vi "create_folder_general-SD.vi"(2 "error in (no error)":errorcluster, 3 "save Radio Buttons":enum32{"Automatic", "User-def"}(ring), 4 "Name":string) -> (0 "error out":errorcluster, 1 "appended path":path)   [LabVIEW 2020]
uses:
  globalVarSD.vi
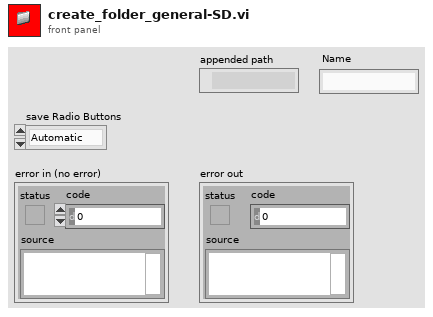
[diagram p1: front panel]
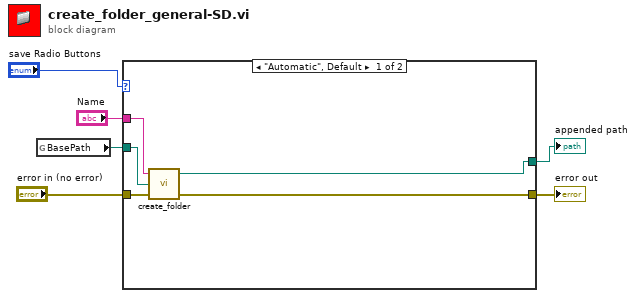
[diagram p0: block diagram]
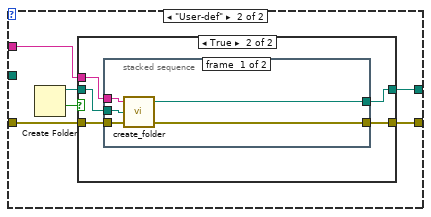
[diagram p2: hidden frame]
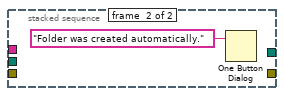
[diagram p4: hidden frame]
diagram:
  n1 = global read "globalVarSD.vi" "BasePath"() -> (w1:path)
  n2 = case shown="\"Automatic\", Default" "save Radio Buttons" {
    tunnel: [w11 w14] -> w2
    tunnel: w1 -> [w8 _]
    tunnel: "error in (no error)" -> [w10 w16]
    tunnel: [w9 w15] -> w5
    tunnel: "Name" -> [w7 w12]
    frame "Automatic", Default {
      n3 = call "create_folder.vi"("Name"=w7, "base path"=w8, "error in"=w10) -> ("appended path"=w11:path, "error out"=w9:errorcluster)  [unwired: 5 in]
    }
    frame "User-def" {
      n4 = Create Folder() -> (created path=w13:path, cancelled=w17:bool)  [unwired: 3 in, 1 out]
      n5 = case shown="True" w17 {
        tunnel: w16 -> [w19 w24]
        tunnel: [w19 w23] -> w15
        tunnel: [w18 w22] -> w14
        tunnel: w13 -> [w18 w21]
        tunnel: w12 -> [_ w20]
        frame False {
        }
        frame True {
          n6 = stacked-sequence {
            tunnel: w24 -> [w29 _]
            tunnel: [w28 _] -> w23
            tunnel: [w27 _] -> w22
            tunnel: w21 -> [w26 _]
            tunnel: w20 -> [w25 _]
            frame #0 {
              n7 = call "create_folder.vi"("Name"=w25, "base path"=w26, "error in"=w29) -> ("appended path"=w27:path, "error out"=w28:errorcluster)  [unwired: 5 in]
            }
            frame #1 {
              n8 = One Button Dialog(message="Folder was created automatically.") -> ()  [unwired: 1 in, 1 out]
            }
          }
        }
      }
    }
  }
  "error out" <- w5
  "appended path" <- w2
